vi "Clean Up Name For Plant UML.vi"(11 "Class Name":string) -> (3 "Plant UML Class Name":string)   [LabVIEW 2020]
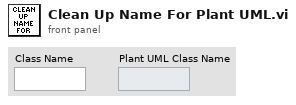
[diagram p1: front panel]
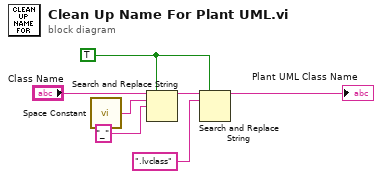
[diagram p0: block diagram]
diagram:
  w3 = TRUE ("replace all? (F)")
  n1 = call <vilib>:"Space Constant.vi"() -> ("String"=w6:string)
  n2 = Search and Replace String(replace all?=w3, input string="Class Name", search string=w6, replace string="_" ("replace string (\"\")")) -> (result string=w4:string)  [unwired: 4 in, 3 out]
  n3 = Search and Replace String(replace all?=w3, input string=w4, search string=".lvclass") -> (result string=→"Plant UML Class Name":string)  [unwired: 5 in, 3 out]
